vi "_Fade Out(I32).vi"(6 "Fade (Exponential)":T1, 8 "error in":errorcluster, 10 "Fade time (ms)":i32, 11 "VI Reference (calling VI)":refnum<vi>) -> (0 "error out":errorcluster, 3 "dup VI Reference":refnum<vi>)   [LabVIEW 2012]
doc: "Produces a \"Fade Out\" on the VI from which a reference has been provided."
uses:
  _fadetype.ctl
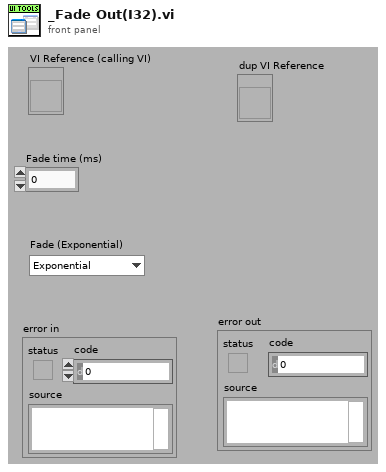
[diagram p1: front panel]
types:
  T1 = typedef "_fadetype.ctl" = enum16{"Exponential", "Linear"}
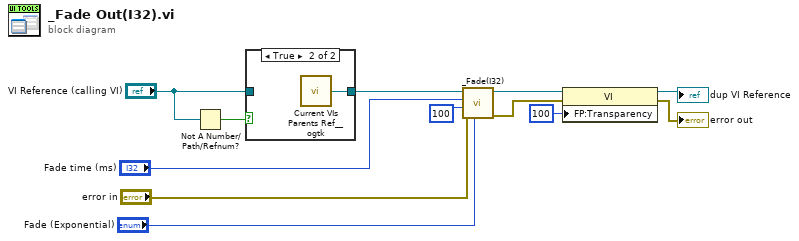
[diagram p0: block diagram]
diagram:
  n1 = Not A Number/Path/Refnum?(number/path/refnum="VI Reference (calling VI)") -> (NaN/Path/Refnum?=w12:bool)
  n2 = case shown="True" w12 {
    tunnel: "VI Reference (calling VI)" -> [w13 _]
    tunnel: [w13 w14] -> w3
    frame False {
    }
    frame True {
      n3 = call <userlib>:"Current VIs Parents Ref__ogtk.vi"() -> ("Calling VI's Reference"=w14:refnum<vi>)  [unwired: 2 out]
    }
  }
  n4 = call "_Fade(I32).vi"("Fade (Exponential)"="Fade (Exponential)", "error in"="error in", "Target Transparency (0)"=u8 100 ("Front Panel Window:Transparency"), "Fade time (ms)"="Fade time (ms)", "VI Reference (calling VI)"=w3) -> ("error out"=w7:errorcluster, "dup VI Reference"=w9:refnum<vi>)  [unwired: 5 out]
  n5 = property class="VI"(reference=w9, error in=w7, "FP:Transparency"=u8 100 ("Front Panel Window:Transparency")) -> (reference out=→"dup VI Reference":refnum<vi>, error out=→"error out":errorcluster)
